vi "16-bit Image to RGB and 8-bit LV 8.6.vi"() -> ()   [LabVIEW 2017]
uses:
  <vilib>/vision/NI_Vision_Development_Module.lvlib
panel:
  out "8-bit":T1(plugin-control)
  out "RGB Image":T1(plugin-control)
  out "Original Image":T1(plugin-control)
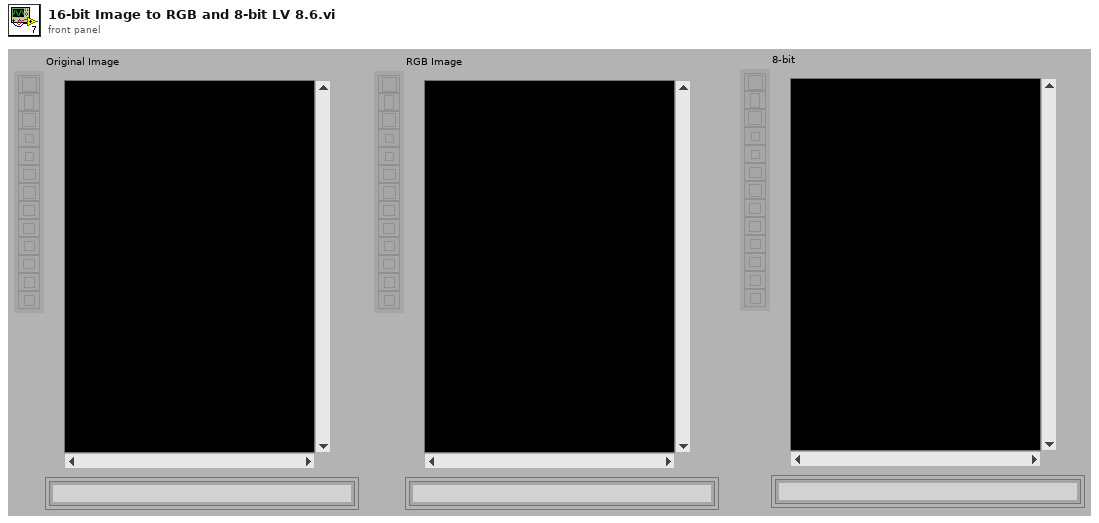
[diagram p1: front panel]
types:
  T1 = typedef "IMAQ Image.ctl" = refnum<image>
  T2 = typedef "Image Type" = u32
  T3 = typedef "AviRefnum.ctl" = refnum<k1>
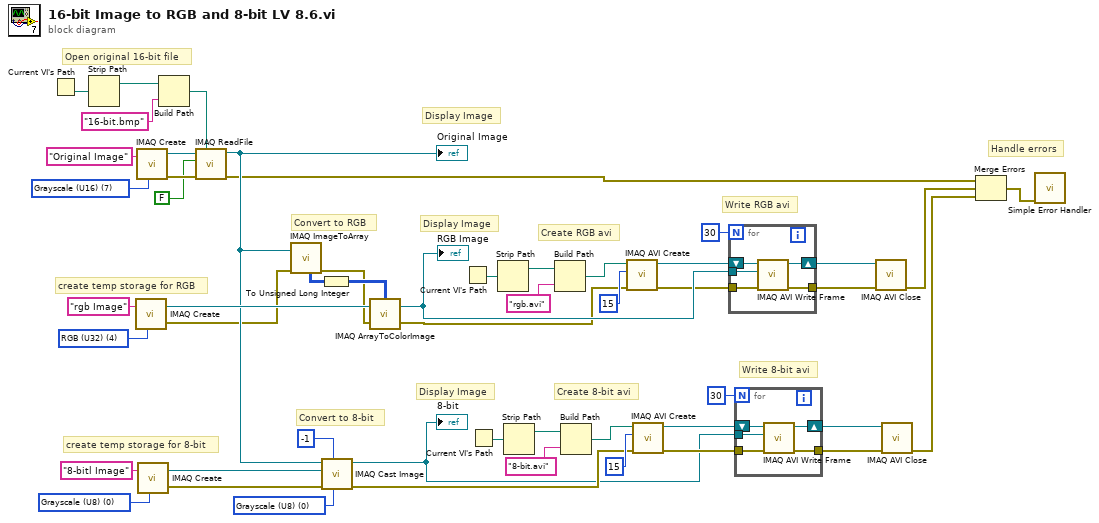
[diagram p0: block diagram]
diagram:
  w33 = T2 0 items=["Grayscale (U8)", "Grayscale (I16)", "Grayscale (SGL)", "Complex (CSG)", "RGB (U32)", "HSL (U32)", "RGB (U64)", "Grayscale (U16)"] ("Image Type")
  w37 = T2 0 items=["Grayscale (U8)", "Grayscale (I16)", "Grayscale (SGL)", "Complex (CSG)", "RGB (U32)", "HSL (U32)", "RGB (U64)", "Grayscale (U16)"] ("Image Type")
  w44 = T2 4 items=["Grayscale (U8)", "Grayscale (I16)", "Grayscale (SGL)", "Complex (CSG)", "RGB (U32)", "HSL (U32)", "RGB (U64)", "Grayscale (U16)"] ("Image Type")
  w49 = T2 7 items=["Grayscale (U8)", "Grayscale (I16)", "Grayscale (SGL)", "Complex (CSG)", "RGB (U32)", "HSL (U32)", "RGB (U64)", "Grayscale (U16)"] ("Image Type")
  # "Handle errors"
  # "Write 8-bit avi"
  # "Write RGB avi"
  # "Display Image"
  # "Display Image"
  # "Display Image"
  # "Create 8-bit avi"
  # "Create RGB avi"
  # "Convert to 8-bit"
  # "Convert to RGB"
  # "create temp storage for 8-bit"
  # "create temp storage for RGB"
  # "Open original 16-bit file"
  n1 = Current VI's Path() -> (path=w41:path)
  n2 = Strip Path(path=w41) -> (stripped path=w40:path)  [unwired: 1 out]
  n3 = call "IMAQ Create"("Image Name"="rgb Image", "Image Type"=w44) -> ("New Image"=w42:T1, "error out"=w22:errorcluster)  [unwired: 2 in, 1 out]
  n4 = call "IMAQ Create"("Image Name"="Original Image", "Image Type"=w49) -> ("New Image"=w51:T1, "error out"=w50:errorcluster)  [unwired: 2 in, 1 out]
  n5 = call "IMAQ Create"("Image Name"="8-bitl Image", "Image Type"=w37) -> ("New Image"=w35:T1, "error out"=w6:errorcluster)  [unwired: 2 in, 1 out]
  n6 = Build Path(base path=w40, name or relative path="16-bit.bmp") -> (appended path=w38:path)
  n7 = call "IMAQ ReadFile"("File Path"=w38, "error in (no error)"=w50, "Load Color Palette? (No)"=FALSE, "Image"=w51) -> ("error out"=w4:errorcluster, "Image Out"=w34:T1)  [unwired: 1 in, 5 out]
  "Original Image" <- w34
  n8 = call "IMAQ ImageToArray"("error in (no error)"=w22, "Image"=w34) -> ("Image Pixels (U16)"=w46:u16[][], "error out"=w21:errorcluster)  [unwired: 1 in, 4 out]
  n9 = To Unsigned Long Integer(number=w46) -> (unsigned 32bit integer=w43:u32[][])
  n10 = call "IMAQ Cast Image"("Image Type"=w33, "# Shifts"=-1, "error in (no error)"=w6, "Image Dst"=w35, "Image Src"=w34) -> ("error out"=w7:errorcluster, "Image Dst Out"=w5:T1)  [unwired: 1 in, 4 out]
  "8-bit" <- w5
  n11 = call "IMAQ ArrayToColorImage"("Image Pixels (U32)"=w43, "Image"=w42, "error in (no error)"=w21) -> ("Image Out"=w23:T1, "error out"=w20:errorcluster)  [unwired: 1 in, 1 out]
  "RGB Image" <- w23
  n12 = Current VI's Path() -> (path=w28:path)
  n13 = Current VI's Path() -> (path=w11:path)
  n14 = Strip Path(path=w28) -> (stripped path=w29:path)  [unwired: 1 out]
  n15 = Strip Path(path=w11) -> (stripped path=w10:path)  [unwired: 1 out]
  n16 = Build Path(base path=w29, name or relative path="rgb.avi") -> (appended path=w27:path)
  n17 = Build Path(base path=w10, name or relative path="8-bit.avi") -> (appended path=w12:path)
  n18 = call "IMAQ AVI Create"("error in (no error)"=w20, "Frames Per Second"=u32 15, "AVI Path"=w27) -> ("error out"=w19:errorcluster, "Avi Refnum"=w25:T3)  [unwired: 4 in, 3 out]
  n19 = call "IMAQ AVI Create"("error in (no error)"=w7, "Frames Per Second"=u32 15, "AVI Path"=w12) -> ("error out"=w16:errorcluster, "Avi Refnum"=w14:T3)  [unwired: 4 in, 3 out]
  n20 = for {
    N: 30 -> [_]
    shift-right: [w55] -> w24
    shift-left: w25 -> [w56]
    tunnel: w23 -> [w54]
    tunnel: w19 -> [w53]
    tunnel: [w52] -> w18
    n21 = call "IMAQ AVI Write Frame"("error in (no error)"=w53, "Image"=w54, "Avi Refnum"=w56) -> ("error out"=w52:errorcluster, "Avi Refnum (duplicate)"=w55:T3)  [unwired: 1 in, 6 out]
  }
  n22 = for {
    N: 30 -> [_]
    shift-right: [w60] -> w15
    shift-left: w14 -> [w61]
    tunnel: w5 -> [w59]
    tunnel: w16 -> [w58]
    tunnel: [w57] -> w17
    n23 = call "IMAQ AVI Write Frame"("error in (no error)"=w58, "Image"=w59, "Avi Refnum"=w61) -> ("error out"=w57:errorcluster, "Avi Refnum (duplicate)"=w60:T3)  [unwired: 1 in, 6 out]
  }
  n24 = call "IMAQ AVI Close"("error in (no error)"=w18, "Avi Refnum"=w24) -> ("error out"=w3:errorcluster)  [unwired: 9 out]
  n25 = call "IMAQ AVI Close"("error in (no error)"=w17, "Avi Refnum"=w15) -> ("error out"=w2:errorcluster)  [unwired: 9 out]
  n26 = Merge Errors(w4, w3, w2) -> (w1:errorcluster)
  n27 = call <vilib>:"Simple Error Handler.vi"("error in (no error)"=w1) -> ()  [unwired: 1 in, 8 out]
